vi "Set Up.vi"() -> ()   [LabVIEW 2017]
panel:
  out "useLCD":bool[][](array[boolean])=[[FALSE, FALSE, FALSE, FALSE, FALSE], [TRUE, TRUE, TRUE, TRUE, FALSE], [TRUE, TRUE, TRUE, TRUE, FALSE], [TRUE, TRUE, TRUE, TRUE, FALSE], [TRUE, FALSE, FALSE, FALSE, FALSE], [TRUE, FALSE, FALSE, FALSE, FALSE], [FALSE, FALSE, FALSE, FALSE, FALSE]]
  out "usePCspec":bool[][](array[boolean])=[[TRUE, TRUE, TRUE, TRUE, TRUE], [TRUE, TRUE, TRUE, TRUE, FALSE], [TRUE, TRUE, TRUE, TRUE, FALSE], [TRUE, TRUE, TRUE, TRUE, FALSE], [FALSE, FALSE, TRUE, FALSE, FALSE], [FALSE, FALSE, FALSE, FALSE, FALSE], [FALSE, FALSE, FALSE, FALSE, FALSE]]
  out "ttimeadjust":dbl[][](array[numeric])=[[1.0, 1.0, 1.0, 1.0, 1.0], [2.0, 2.0, 2.0, 2.0, 1.0], [2.0, 2.0, 2.0, 2.0, 0.0], [2.0, 2.0, 2.0, 2.0, 0.0], [2.0, 1.0, 1.0, 1.0, 0.0], [2.0, 1.0, 1.0, 1.0, 0.0], [1.0, 1.0, 1.0, 1.0, 0.0], [1.0, 1.0, 1.0, 1.0, 1.0], [1.0, 1.0, 1.0, 1.0, 1.0]]
  in  "timeest":cluster{"m":dbl, "b":dbl[unit]}[][](array[cluster])=[[{"m"=1.1, "b"=0.6}, {"m"=1.0, "b"=0.1}, {"m"=1.0, "b"=0.3}, {"m"=1.0, "b"=0.0}, {"m"=1.0, "b"=0.0}], [{"m"=1.1, "b"=0.6}, {"m"=1.0, "b"=0.1}, {"m"=1.0, "b"=0.3}, {"m"=1.0, "b"=0.0}, {"m"=1.0, "b"=0.0}], [{"m"=1.1, "b"=0.6}, {"m"=1.0, "b"=0.1}, {"m"=1.0, "b"=0.3}, {"m"=1.0, "b"=0.0}, {"m"=1.0, "b"=0.0}], [{"m"=1.1, "b"=0.6}, {"m"=1.0, "b"=0.1}, {"m"=1.0, "b"=0.3}, {"m"=1.0, "b"=0.0}, {"m"=1.0, "b"=0.0}], [{"m"=1.1, "b"=0.8}, {"m"=0.0, "b"=0.0}, {"m"=1.0, "b"=0.3}, {"m"=1.0, "b"=0.0}, {"m"=1.0, "b"=0.0}], [{"m"=1.1, "b"=0.8}, {"m"=0.0, "b"=0.0}, {"m"=0.0, "b"=0.0}, {"m"=1.0, "b"=0.0}, {"m"=1.0, "b"=0.0}], [{"m"=1.1, "b"=0.8}, {"m"=0.0, "b"=0.0}, {"m"=0.0, "b"=0.0}, {"m"=0.0, "b"=0.0}, {"m"=1.0, "b"=0.0}], [{"m"=1.1, "b"=0.8}, {"m"=0.0, "b"=0.0}, {"m"=0.0, "b"=0.0}, {"m"=1.0, "b"=0.0}, {"m"=1.0, "b"=0.0}], [{"m"=0.0, "b"=0.0}, {"m"=0.0, "b"=0.0}, {"m"=0.0, "b"=0.0}, {"m"=0.0, "b"=0.0}, {"m"=1.0, "b"=0.0}]]
  out "polarization":string[][](array[string])=[["pol", "pol", "pol", "pol", "pol"], ["pol", "pol", "pol", "pol", "ld"], ["opt,therm", "opt,therm", "opt,therm", "opt,therm", "none"], ["opt,therm", "opt,therm", "opt,therm", "opt,therm", "none"], ["opt,therm", "none", "none", "none", "none"], ["opt,therm", "none", "none", "ld", "none"], ["ld", "none", "none", "ld", "none"], ["ld", "none", "none", "none", "none"], ["none", "none", "none", "none", "none"]]
  out "gating":bool[][](array[boolean])=[[TRUE, TRUE, TRUE, TRUE, TRUE], [FALSE, FALSE, FALSE, FALSE, FALSE], [TRUE, TRUE, TRUE, TRUE, FALSE], [TRUE, TRUE, TRUE, TRUE, FALSE], [TRUE, FALSE, FALSE, FALSE, FALSE], [TRUE, FALSE, FALSE, FALSE, FALSE], [FALSE, FALSE, FALSE, FALSE, FALSE], [FALSE, FALSE, FALSE, FALSE, FALSE], [FALSE, FALSE, FALSE, FALSE, FALSE]]
  out "instrneeded":string[][](array[string])=[["pc,sp,pg", "pc,sp,pg", "pc,sp", "pc,sp,mg", "pc,sp,fg,mg"], ["pc,lc,sp,pg", "pc,lc,sp,pg", "pc,lc,sp", "pc,lc,sp,mg", "ld,fg,mg"], ["pc,lc,sp,pg", "pc,lc,sp,pg", "pc,lc,sp", "pc,lc,sp,mg", "none"], ["pc,lc,sp,pg", "pc,lc,sp,pg", "pc,lc,sp", "pc,lc,sp,mg", "none"], ["pc,lc,sp,pg", "none", "pc,sp", "pc,sp,mg", "none"], ["pc,lc,sp,pg", "none", "none", "ld,mg", "none"], ["mg,pg,ld", "none", "none", "ld,mg", "none"], ["mg,pg,ld", "none", "none", "none", "none"], ["none", "none", "none", "none", "none"]]
  out "setup":string[][](array[string])=[["2 Ch PC", "2 Ch PC", "2 Ch PC", "2 Ch PC", "2 Ch PC"], ["2 Ch PC", "2 Ch PC", "2 Ch PC", "2 Ch PC", "LD"], ["4 Ch PC", "4 Ch PC", "4 Ch PC", "4 Ch PC", "none"], ["4 Ch PC", "4 Ch PC", "4 Ch PC", "4 Ch PC", "none"], ["Echo PC", "none", "1 Ch PC", "1 Ch PC", "none"], ["Echo PC", "none", "1 Ch PC", "LD", "none"], ["Echo KR", "none", "none", "LD", "none"], ["LD", "none", "none", "none", "none"], ["none", "none", "none", "none", "none"]]
  out "labels":T1(array[cluster])=[{"Data Column Headings"=["CPS"], "Primary Plot Labels"=["CPS"], "Secondary Plot Labels"=[], "Tag"="1 Ch PC", "Y-axis"="Light Intensity (CPS)", "Total # Columns (incl. X-var)"=2.0, "Index of first Secondary\nColumn (from 0)"=0.0, "# Secondary Columns"=0.0, "# Data Columns (deprecated)"=1.0, "# Data Columns"=1.0}, {"Data Column Headings"=["Ch A", "Ch B", "Average", "Polarization"], "Primary Plot Labels"=["Channel A", "Channel B"], "Secondary Plot Labels"=["Polarization"], "Tag"="2 Ch PC", "Y-axis"="Light Intensity (CPS)", "Total # Columns (incl. X-var)"=5.0, "Index of first Secondary\nColumn (from 0)"=3.0, "# Secondary Columns"=1.0, "# Data Columns (deprecated)"=3.0, "# Data Columns"=2.0}, {"Data Column Headings"=["1/4D,1/4E", "1/4D,3/4E", "3/4D,1/4E", "3/4D,3/4E", "Average", "Thermal Pol", "Optical Pol", "1/4 Det", "3/4 Det", "ChA Therm", "ChB Therm"], "Primary Plot Labels"=["1/4D,1/4E", "1/4D,3/4E", "3/4D,1/4E", "3/4D,3/4E"], "Secondary Plot Labels"=["Thermal Pol", "Optical Pol"], "Tag"="4 Ch PC", "Y-axis"="Light Intensity (CPS)", "Total # Columns (incl. X-var)"=12.0, "Index of first Secondary\nColumn (from 0)"=6.0, "# Secondary Columns"=2.0, "# Data Columns (deprecated)"=9.0, "# Data Columns"=4.0}, {"Data Column Headings"=["1/4D,1/4E", "3/4D,1/4E", "1/4D,3/4E", "3/4D,3/4E", "Average", "Thermal Pol", "Optical Pol", "1/4 Det", "3/4 Det", "ChA Therm", "ChB Therm"], "Primary Plot Labels"=["1/4D,1/4E", "3/4D,1/4E", "1/4D,3/4E", "3/4D,3/4E"], "Secondary Plot Labels"=["Thermal Pol", "Optical Pol"], "Tag"="NA", "Y-axis"="Light Intensity (CPS)", "Total # Columns (incl. X-var)"=12.0, "Index of first Secondary\nColumn (from 0)"=6.0, "# Secondary Columns"=2.0, "# Data Columns (deprecated)"=9.0, "# Data Columns"=4.0}, {"Data Column Headings"=["Lockin Ch 1", "Lockin Ch 2"], "Primary Plot Labels"=["Lockin Ch 1", "Lockin Ch 2"], "Secondary Plot Labels"=["None"], "Tag"="LD", "Y-axis"="Lock-in Signal (V)", "Total # Columns (incl. X-var)"=3.0, "Index of first Secondary\nColumn (from 0)"=3.0, "# Secondary Columns"=0.0, "# Data Columns (deprecated)"=2.0, "# Data Columns"=3.0}, {"Data Column Headings"=["Lockin Ch 1", "Lockin Ch 2"], "Primary Plot Labels"=["Lockin Ch 1", "Lockin Ch 2"], "Secondary Plot Labels"=["None"], "Tag"="Echo KR", "Y-axis"="Lock-in Signal (V)", "Total # Columns (incl. X-var)"=3.0, "Index of first Secondary\nColumn (from 0)"=3.0, "# Secondary Columns"=0.0, "# Data Columns (deprecated)"=2.0, "# Data Columns"=3.0}, {"Data Column Headings"=["1/4D,1/4E", "1/4D,3/4E", "3/4D,1/4E", "3/4D,3/4E", "Average", "Thermal Pol", "Optical Pol", "1/4 Det", "3/4 Det", "ChA Therm", "ChB Therm"], "Primary Plot Labels"=["1/4D,1/4E", "1/4D,3/4E", "3/4D,1/4E", "3/4D,3/4E"], "Secondary Plot Labels"=["Thermal Pol", "Optical Pol"], "Tag"="Echo PC", "Y-axis"="Light Intensity (CPS)", "Total # Columns (incl. X-var)"=12.0, "Index of first Secondary\nColumn (from 0)"=6.0, "# Secondary Columns"=2.0, "# Data Columns (deprecated)"=9.0, "# Data Columns"=4.0}, {"Data Column Headings"=["Ch A", "Ch B", "Average", "Polarization"], "Primary Plot Labels"=["Ch A", "Ch B"], "Secondary Plot Labels"=[], "Tag"="KR PC", "Y-axis"="CPS", "Total # Columns (incl. X-var)"=5.0, "Index of first Secondary\nColumn (from 0)"=3.0, "# Secondary Columns"=2.0, "# Data Columns (deprecated)"=3.0, "# Data Columns"=2.0}, {"Data Column Headings"=["Ch A", "Ch B"], "Primary Plot Labels"=["Ch A", "Ch B"], "Secondary Plot Labels"=["Polarization"], "Tag"="temp", "Y-axis"="CPS", "Total # Columns (incl. X-var)"=4.0, "Index of first Secondary\nColumn (from 0)"=3.0, "# Secondary Columns"=2.0, "# Data Columns (deprecated)"=3.0, "# Data Columns"=2.0}]
  out "setupscan":T2(array[cluster])=[{"name"="Wait Time", "xunit"="ns", "xaxis"="Wait Time (ns)"}, {"name"="Pulse Width", "xunit"="ns", "xaxis"="Pulse Width (ns)"}, {"name"="Wavelength", "xunit"="nm", "xaxis"="Wavelength (nm)"}, {"name"="Magnetic Field", "xunit"="T", "xaxis"="Magnetic Field (T)"}, {"name"="rf Scan", "xunit"="MHz", "xaxis"="rf (MHz)"}]
  # "total cols does include the x-value col"
  # "exp type"
  # "wait time"
  # "pulse\nwidth"
  # "wave"
  # "magfield"
  # "rf scan"
  # "exp mode"
  # "scan type"
  # "SP\nPG\nLC\nPC\nLD\nMG"
  # "List all instruments needed!!"
  # "Wait Time"
  # "Pulse Width"
  # "Wavelength"
  # "Magnetic Field"
  # "rf scan"
  # "exp modes go as follows:"
  # "PEM\nLCD\nPEM-LCD\nLCD-PEM\nEcho P-L\nEcho L-P\nEcho KR\nLock-in"
  # "PEM\nLCD\nPEM-LCD\nLCD-PEM"
  # "PEM\nLCD\nPEM-LCD\nLCD-PEM\nNo Ret."
  # "PEM\nLCD\nPEM-LCD\nLCD-PEM\nNo Ret.\nStep LD\nCont. LD"
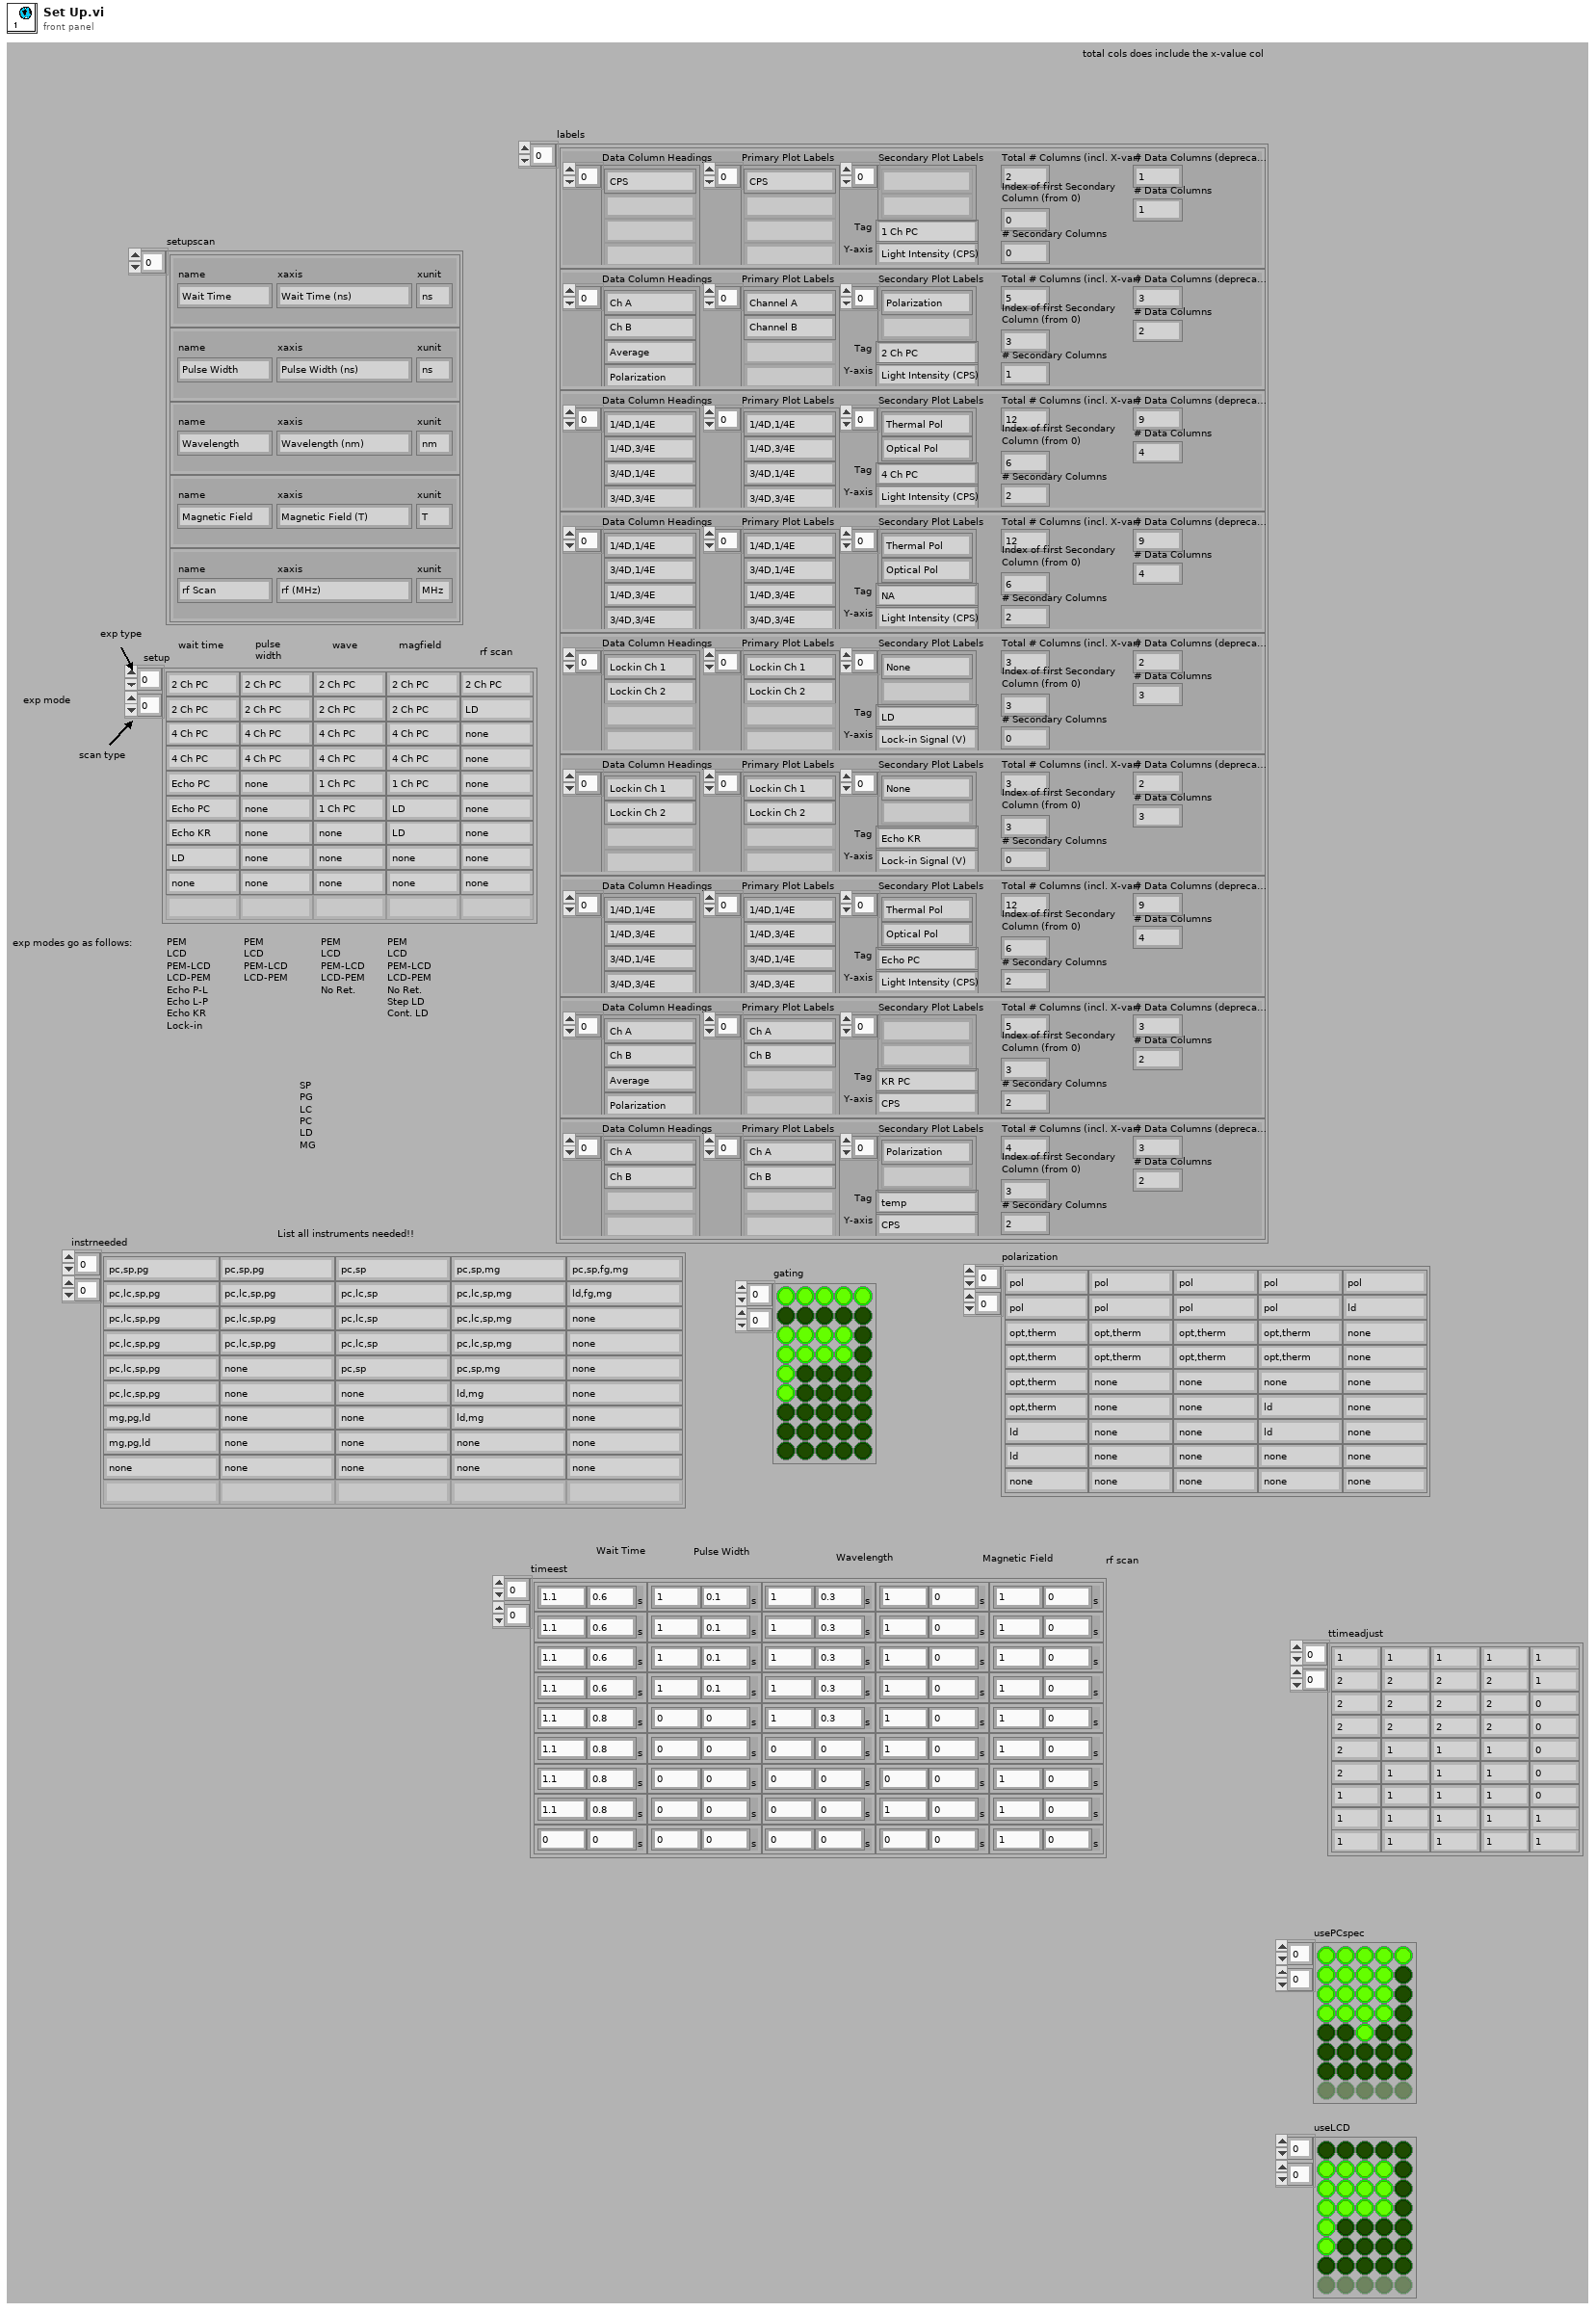
[diagram p1: front panel]
types:
  T1 = cluster{"Data Column Headings":string[], "Primary Plot Labels":string[], "Secondary Plot Labels":string[], "Tag":string, "Y-axis":string, "Total # Columns (incl. X-var)":dbl, "Index of first Secondary\nColumn (from 0)":dbl, "# Secondary Columns":dbl, "# Data Columns (deprecated)":dbl, "# Data Columns":dbl}[]
  T2 = cluster{"name":string, "xunit":string, "xaxis":string}[]
diagram:
